vi "Read Element of Columns.vi"(10 "index":i32, 11 "Series in":refnum<class "Series.lvclass">) -> (2 "?":string, 3 "Series out":refnum<class "Series.lvclass">)   [LabVIEW 2018, in "InfluxDB Client.lvlib" / "Series.lvclass"]
uses:
  Series.lvclass
  Series.lvclass/Series.ctl
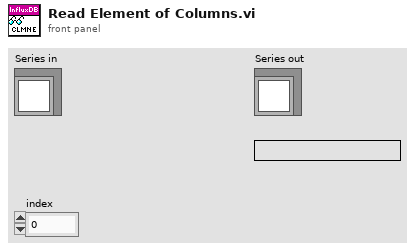
[diagram p1: front panel]
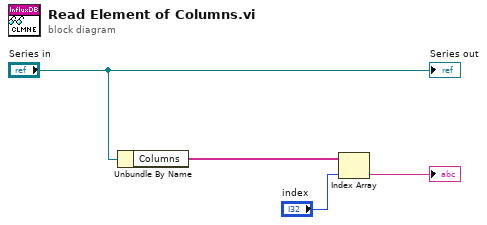
[diagram p0: block diagram]
diagram:
  n1 = Unbundle By Name("Series in") -> ("Columns"=w2:string[])
  n2 = Index Array(array=w2, index="index") -> (element=→"?":string)
  "Series out" <- "Series in"
